vi "Init Osciloscope.vi"(8 "error in":errorcluster, 10 "Initialize--cluster":T1={"Serial Configuration"={"Baud Rate"=9600, "Parity"=0, "Stop Bits"=10, "Flow Control"=2}, "ID Query? (T: Yes)"=TRUE, "Reset? (T: Yes)"=TRUE} {"Serial Configuration"."Flow Control" items=["None", "XON/XOFF", "RTS/CTS", "XON/XOFF & RTS/CTS", "DTR/DSR", "XON/XOFF & DTR/DSR"]; "Serial Configuration"."Stop Bits" items=["1.0"=10, "1.5"=15, "2.0"=20]; "Serial Configuration"."Parity" items=["None", "Odd", "Even", "Mark", "Space"]; "Serial Configuration"."Baud Rate" items=["300"=300, "600"=600, "1200"=1200, "2400"=2400, "4800"=4800, "9600"=9600, "19200"=19200]}, 11 "Module ID":i32=-1) -> (0 "error out":errorcluster)   [LabVIEW 2020, in "Osciloscope.lvlib"]
doc: "_____\nCreated using DQMH Event Scripter 6.0.0.122."
uses:
  Osciloscope.lvlib
  TypeDefs/InitializeOsciloscope--cluster.ctl
  Init Osciloscope Argument--cluster.ctl
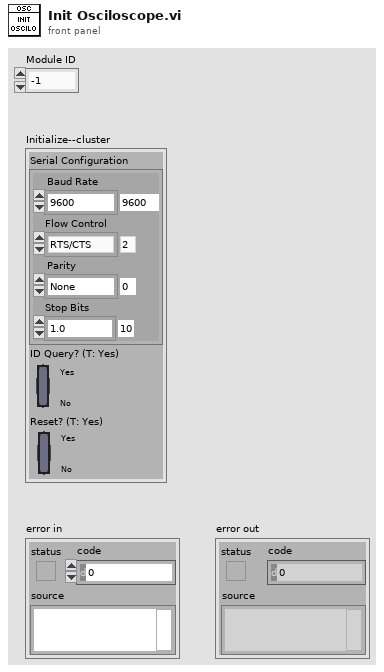
[diagram p1: front panel]
types:
  T1 = typedef "InitializeOsciloscope--cluster.ctl" = cluster{"Serial Configuration":cluster{"Baud Rate":u32, "Parity":u16, "Stop Bits":u16, "Flow Control":u16}, "ID Query? (T: Yes)":bool, "Reset? (T: Yes)":bool}
  T2 = typedef "Osciloscope.lvlib/Init Osciloscope Argument--cluster.ctl" = cluster{"Module ID":i32, "Boolean":bool, "Initialize--cluster":T1}
  T3 = typedef "Osciloscope.lvlib/Request Events--cluster.ctl" = cluster{"Stop Module":refnum<user-event>, "Show Panel":refnum<user-event>, "Hide Panel":refnum<user-event>, "Show Diagram":refnum<user-event>, "Get Module Execution Status":refnum<user-event>, "Set Com Port":refnum<user-event>, "Inizializate":refnum<user-event>, "Init Osciloscope":refnum<user-event>, "Close Osciloscope":refnum<user-event>, "Auto Setup Osciloscope":refnum<user-event>, "Configure Channel":refnum<user-event>, "Reset Osciloscope":refnum<user-event>, "Read Waveform Osciloscope":refnum<user-event>, "Read Measurement Osciloscope":refnum<user-event>, "Read 2 Measurement Channels Osciloscope":refnum<user-event>}
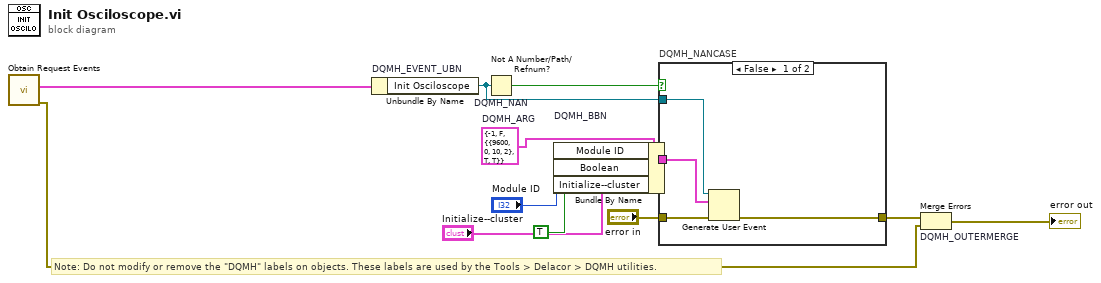
[diagram p0: block diagram]
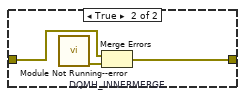
[diagram p2: hidden frame]
diagram:
  w6 = T2 {"Module ID"=-1, "Boolean"=FALSE, "Initialize--cluster"={"Serial Configuration"={"Baud Rate"=9600, "Parity"=0, "Stop Bits"=10, "Flow Control"=2}, "ID Query? (T: Yes)"=TRUE, "Reset? (T: Yes)"=TRUE}}  # DQMH_ARG
  # "Note: Do not modify or remove the \"DQMH\" labels on objects. These labels are used by the Tools > Delacor > DQMH utilities."
  n1 = call "Obtain Request Events.vi"() -> ("error out"=w3:errorcluster, "Osciloscope Request Events"=w2:T3)  [unwired: 10 in]
  n2 = Unbundle By Name "DQMH_EVENT_UBN"(w2) -> ("Init Osciloscope"=w8:refnum<user-event>)
  n3 = Not A Number/Path/Refnum? "DQMH_NAN"(number/path/refnum=w8) -> (NaN/Path/Refnum?=w9:bool)
  n4 = Bundle By Name "DQMH_BBN"(cluster=w6, "Module ID"="Module ID", "Boolean"=TRUE, "Initialize--cluster"="Initialize--cluster") -> (w10:T2)
  n5 = case "DQMH_NANCASE" shown="False" w9 {
    tunnel: "error in" -> [w16 w19]
    tunnel: [w15 w18] -> w7
    tunnel: w8 -> [w14 _]
    tunnel: w10 -> [w13 _]
    frame False {
      n6 = Generate User Event(user event=w14, event data cluster=w13, error in=w16) -> (error out=w15:errorcluster)  [unwired: 1 in, 1 out]
    }
    frame True {
      n7 = call "Module Not Running--error.vi"() -> ("error out"=w17:errorcluster)  [unwired: 11 in]
      n8 = Merge Errors "DQMH_INNERMERGE"(w19, w17) -> (w18:errorcluster)
    }
  }
  n9 = Merge Errors "DQMH_OUTERMERGE"(w7, w3) -> (→"error out":errorcluster)
